vi "FormatIntoString.vi"(1 "System Pos":string[](array[string]), 2 "System Status":string[](array[string])) -> (0 "String out":string)   [LabVIEW 2015]
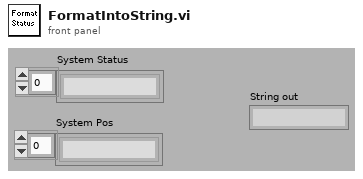
[diagram p1: front panel]
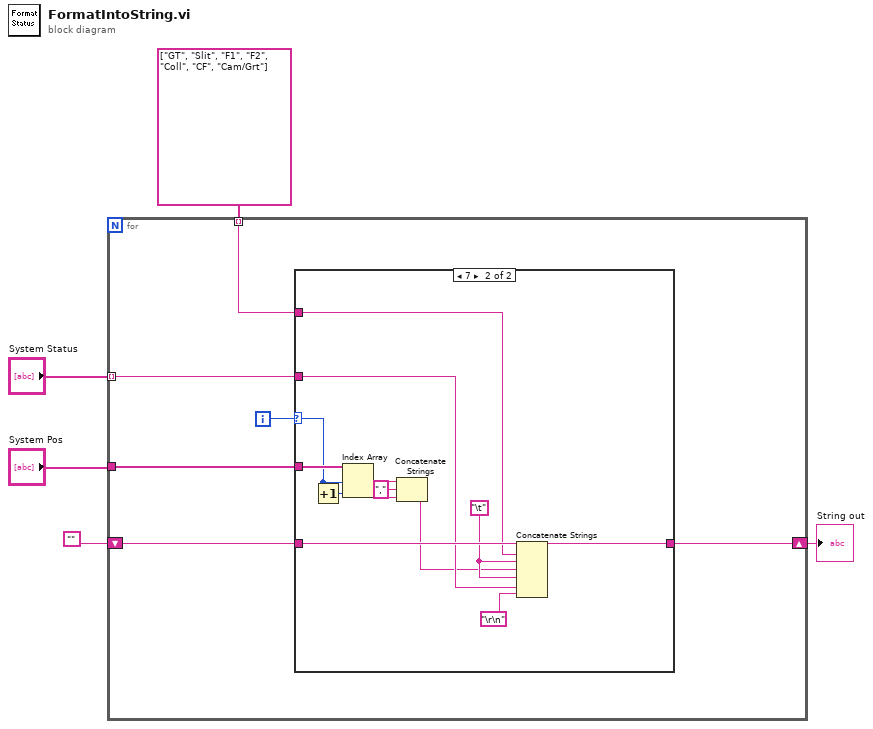
[diagram p0: block diagram]
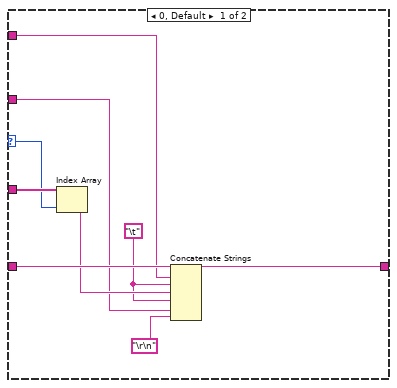
[diagram p2: hidden frame]
diagram:
  n1 = for {
    shift-right: [w6] -> w1
    shift-left: "" -> [w10]
    tunnel: string[] ["GT", "Slit", "F1", "F2", "Coll", "CF", "Cam/Grt"] -> [w11] mode=indexing
    tunnel: "System Pos" -> [w7]
    tunnel: "System Status" -> [w8] mode=indexing
    i -> [w9]
    n2 = case shown="7" w9 {
      selector: w9 -> [w17 w22]
      tunnel: w11 -> [w19 w32]
      tunnel: w10 -> [w20 w33]
      tunnel: w8 -> [w14 w29]
      tunnel: w7 -> [w18 w31]
      tunnel: [w13 w28] -> w6
      frame 0, Default {
        w15 = "\t"
        n3 = Index Array(array=w18, index=w17) -> (element=w16:string)
        n4 = Concatenate Strings(w20, w19, w15, w16, w15, w14, "\r\n") -> (w13:string)
      }
      frame 7 {
        w30 = "\t"
        n5 = Increment(x=w22) -> (x+1=w21:i32)
        n6 = Index Array(array=w31, index #1=w22, index #2=w21) -> (element #1=w27:string, element #2=w26:string)
        n7 = Concatenate Strings(w27, "," ("string"), w26) -> (w24:string)
        n8 = Concatenate Strings(w33, w32, w30, w24, w30, w29, "\r\n") -> (w28:string)
      }
    }
  }
  "String out" <- w1
